vi "Core.vi"(10 "Class Return Notifier":refnum<notifier>, 11 "Engine in":refnum<class "Engine.lvclass">) -> ()   [LabVIEW 2024, in "GLF.lvlib" / "Engine.lvclass"]
doc: "<B>Summary</B>\nThe GLF main process handling SDL events and clients commands."
uses:
  Engine.lvclass
  IAmGLF/IAmGLF.lvclass
  Engine.lvclass/Engine.ctl
  <vilib>/Saukko/LV SDL3/Sources/SDL3/Timer/GetTicks.vi
  <vilib>/Saukko/LV SDL3/Sources/SDL3/Events/PollEvent.vi
  <vilib>/Saukko/LV SDL3/Sources/SDL3/Events/Unflatten-EventType.vi
  <vilib>/Saukko/LV SDL3/Sources/SDL3/Events/ShouldClose.vi
  QuitOnLastWindowClosed-Get.vi
  Core-DequeueCommands.vi/c534fc45-f9c2-42cc-8e01-6a6c0b1517e4.vi
  <vilib>/Saukko/LV SDL3/Sources/SDL3/Timer/Delay.vi
  QuitOnLastWindowClosed-Get.vi/a1934f40-8091-4efc-9cde-54247e41822d.vi
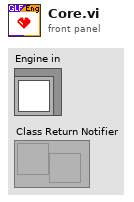
[diagram p1: front panel]
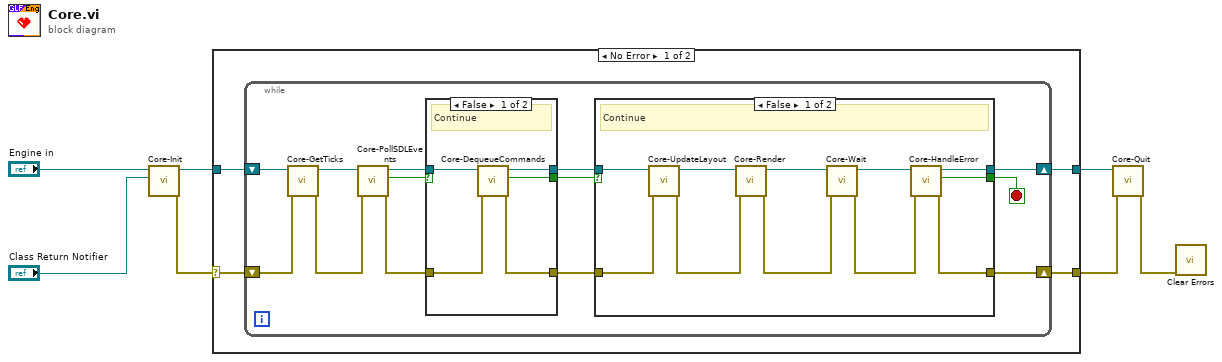
[diagram p0: block diagram]
diagram:
  n1 = call "Core-Init.vi"("Class Return Notifier"="Class Return Notifier", "Engine in"="Engine in") -> ("error out"=w5:errorcluster, "Engine out"=w6:refnum<class "Engine.lvclass">)  [unwired: 8 in]
  n2 = case shown="No Error" w5 {
    selector: w5 -> [w10 w48]
    tunnel: w6 -> [w11 w47]
    tunnel: [w9 w47] -> w4
    tunnel: [w8 w48] -> w3
    frame No Error {
      n3 = while {
        shift-right: [w19] -> w9
        shift-left: w11 -> [w24]
        shift-right: [w17] -> w8
        shift-left: w10 -> [w14]
        stop <- w12 stop-if-true
        n4 = call "Core-GetTicks.vi"("error in (no error)"=w14, "Engine in"=w24) -> ("error out"=w13:errorcluster, "Engine out"=w15:refnum<class "Engine.lvclass">)  [unwired: 8 in]
        n5 = call "Core-PollSDLEvents.vi"("error in (no error)"=w13, "Engine in"=w15) -> ("error out"=w22:errorcluster, "Quit?"=w21:bool, "Engine out"=w23:refnum<class "Engine.lvclass">)  [unwired: 7 in]
        n6 = case shown="False" w21 {
          selector: w21 -> [_ w44]
          tunnel: w23 -> [w43 w46]
          tunnel: w22 -> [w42 w45]
          tunnel: [w41 w45] -> w18
          tunnel: [w40 w46] -> w20
          tunnel: [w39 w44] -> w16
          frame False {
            # "Continue"
            n7 = call "Core-DequeueCommands.vi"("error in (no error)"=w42, "Engine in"=w43) -> ("error out"=w41:errorcluster, "Quit?"=w39:bool, "Engine out"=w40:refnum<class "Engine.lvclass">)  [unwired: 7 in]
          }
          frame True {
            # "Quit"
          }
        }
        n8 = case shown="False" w16 {
          selector: w16 -> [_ w36]
          tunnel: w20 -> [w34 w38]
          tunnel: [w28 w38] -> w19
          tunnel: w18 -> [w29 w37]
          tunnel: [w26 w37] -> w17
          tunnel: [w25 w36] -> w12
          frame False {
            # "Continue"
            n9 = call "Core-UpdateLayout.vi"("error in (no error)"=w29, "Engine in"=w34) -> ("error out"=w30:errorcluster, "Engine out"=w31:refnum<class "Engine.lvclass">)  [unwired: 8 in]
            n10 = call "Core-Render.vi"("error in (no error)"=w30, "Engine in"=w31) -> ("error out"=w32:errorcluster, "Engine out"=w33:refnum<class "Engine.lvclass">)  [unwired: 8 in]
            n11 = call "Core-Wait.vi"("error in (no error)"=w32, "Engine in"=w33) -> ("error out"=w27:errorcluster, "Engine out"=w35:refnum<class "Engine.lvclass">)  [unwired: 8 in]
            n12 = call "Core-HandleError.vi"("error in (no error)"=w27, "Engine in"=w35) -> ("error out"=w26:errorcluster, "Quit?"=w25:bool, "Engine out"=w28:refnum<class "Engine.lvclass">)  [unwired: 7 in]
          }
          frame True {
            # "Quit"
          }
        }
      }
    }
    frame Error {
    }
  }
  n13 = call "Core-Quit.vi"("error in (no error)"=w3, "Engine in"=w4) -> ("error out"=w2:errorcluster)  [unwired: 8 in, 1 out]
  n14 = call <vilib>:"Clear Errors.vi"("error in (no error)"=w2) -> ()  [unwired: 5 in, 2 out]
